vi "feladat_5.vi"() -> ()   [LabVIEW 2021]
uses:
  <vilib>/measure/NI_MABase.lvlib
panel:
  in  "Slide":i32(slide) scale=0.0..3.0
  out "Waveform Graph":waveform(dbl)(graph)
  in  "Offszet":dbl
  in  "Frekvencia":dbl
  in  "Amlitudó":i32
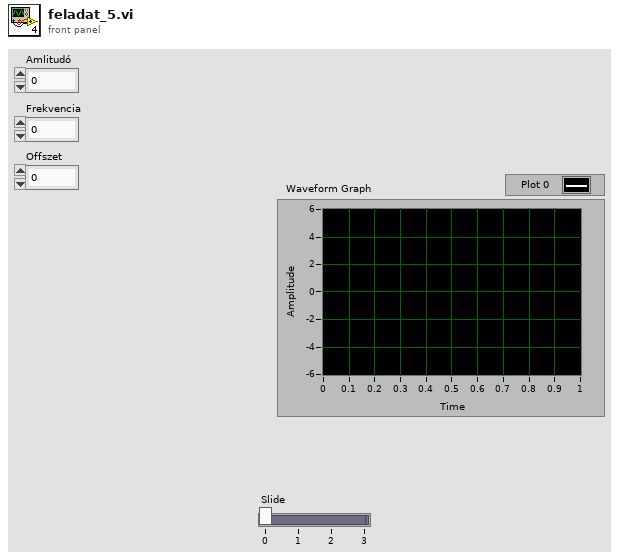
[diagram p1: front panel]
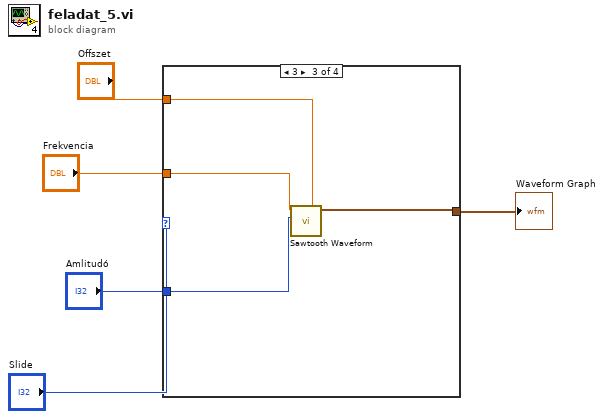
[diagram p0: block diagram]
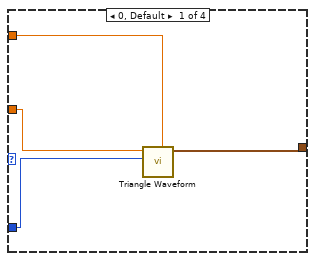
[diagram p2: hidden frame]
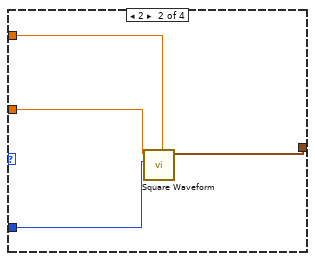
[diagram p3: hidden frame]
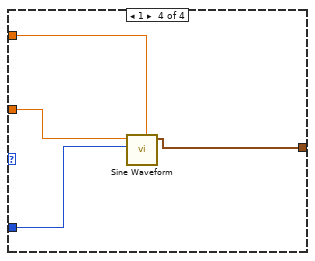
[diagram p4: hidden frame]
diagram:
  n1 = case shown="3" "Slide" {
    tunnel: "Frekvencia" -> [w8 w12 w16 w21]
    tunnel: "Amlitudó" -> [w9 w11 w17 w20]
    tunnel: "Offszet" -> [w7 w13 w15 w19]
    tunnel: [w6 w10 w14 w18] -> w2
    frame 0, Default {
      n2 = call <vilib>:"Triangle Waveform.vi"("offset"=w7, "amplitude"=w9, "frequency"=w8) -> ("signal out"=w6:waveform(dbl))  [unwired: 7 in, 1 out]
    }
    frame 2 {
      n3 = call <vilib>:"Square Waveform.vi"("offset"=w13, "amplitude"=w11, "frequency"=w12) -> ("signal out"=w10:waveform(dbl))  [unwired: 7 in, 1 out]
    }
    frame 3 {
      n4 = call <vilib>:"Sawtooth Waveform.vi"("offset"=w15, "amplitude"=w17, "frequency"=w16) -> ("signal out"=w14:waveform(dbl))  [unwired: 7 in, 1 out]
    }
    frame 1 {
      n5 = call <vilib>:"Sine Waveform.vi"("offset"=w19, "amplitude"=w20, "frequency"=w21) -> ("signal out"=w18:waveform(dbl))  [unwired: 7 in, 1 out]
    }
  }
  "Waveform Graph" <- w2
